vi "svl_Log View for Peak Level (array).vi"(7 "channel info":T1={"sensor sensitivity"=1000.0, "engineering units"=1, "dB reference"=1.0, "custom label"="EU", "weighting filter"=0, "pregain"=0.0} {"pregain" format="%.2f"; "weighting filter" items=["Linear", "A-weighting", "B-weighting", "C-weighting", "ITU-R 468-4", "Dolby", "CCITT", "C-message", "Wb", "Wc", "Wd", "We", "Wf", "Wh", "Wj", "Wk", "Wm", "AES17 20 kHz lowpass", "AES17 40 kHz lowpass", "AES17 20 kHz highpass", "AES17 40 kHz highpass"]; "dB reference" format="%^.1e"; "engineering units" items=["custom..."=0, "V"=1, "A"=21, "C"=30, "pC"=31, "s"=32, "-"=29, "Pa"=2, "N"=20, "g"=3, "m/s^2"=4, "m/s"=5, "m"=6, "mm/s"=12, "mm"=13, "micron/s"=14, "micron"=15, "in/s^2"=7, "in/s"=8, "in"=9, "mil/s"=10, "mil"=11, "rad/s^2"=16, "rad/s"=17, "rad"=18, "deg/s^2"=26, "deg/s"=27, "deg"=28, "RPM"=22, "cycle/s^2"=23, "Hz"=24, "cycle"=25, "strain"=19]; "sensor sensitivity" format="%#_5f"}, 8 "error in (no error)":errorcluster, 10 "dB On (T)":bool=TRUE, 11 "peak level [EU]":dbl[](array[numeric]) format="%.2f") -> (0 "error out":errorcluster, 2 "unit label":string, 3 "peak level [dB EU]":dbl[](array[numeric]) format="%.2f")   [LabVIEW 2017]
uses:
  <vilib>/addons/_NISVFA/_Shared subVIs/Controls/svc_Channel Info.ctl
  <vilib>/addons/_NISVFA/_Shared subVIs/Controls/svc_Engineering Units Text Ring.ctl
  <vilib>/addons/_NISVFA/_Shared subVIs/Controls/svc_Weighting Filter Text Ring.ctl
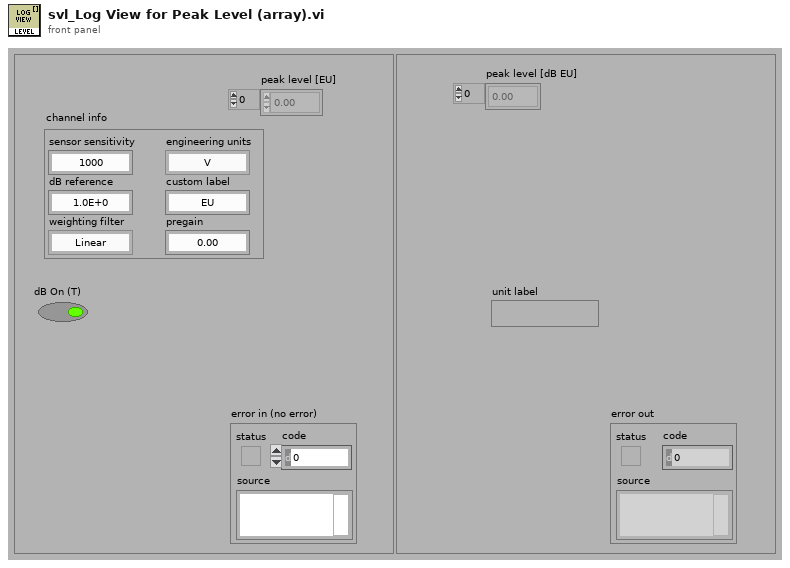
[diagram p1: front panel]
types:
  T1 = typedef "svc_Channel Info.ctl" = cluster{"sensor sensitivity":dbl, "engineering units":T2, "dB reference":dbl, "custom label":string, "weighting filter":T3, "pregain":dbl}
  T2 = typedef "svc_Engineering Units Text Ring.ctl" = u16
  T3 = typedef "svc_Weighting Filter Text Ring.ctl" = u16
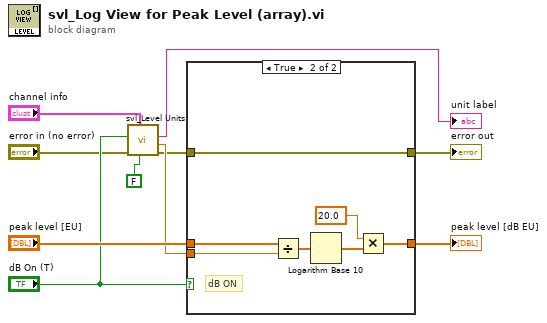
[diagram p0: block diagram]
diagram:
  n1 = call <vilib>:"svl_Level Units.vi"("rms level (T)"=FALSE, "channel info"="channel info", "error in (no error)"="error in (no error)", "dB On (T)"="dB On (T)") -> ("error out"=w2:errorcluster, "dB reference [EU]"=w3:dbl, "unit label"=→"unit label":string)  [unwired: 5 in]
  n2 = case shown="True" "dB On (T)" {
    tunnel: [w11 w19] -> w8
    tunnel: w2 -> [w12 w13]
    tunnel: [w12 w13] -> w10
    tunnel: "peak level [EU]" -> [w11 w18]
    tunnel: w3 -> [_ w14]
    frame False {
      # "dB OFF"
    }
    frame True {
      # "dB ON"
      n3 = Divide(x=w18, y=w14) -> (x/y=w16:dbl[])
      n4 = Logarithm Base 10(1:w16) -> (0:w17:dbl[])
      n5 = Multiply(x=20.0 ("y"), y=w17) -> (x*y=w19:dbl[])
    }
  }
  "peak level [dB EU]" <- w8
  "error out" <- w10
